vi "Color Wheel Controller.vi"(8 "error in":errorcluster) -> ()   [LabVIEW 2019]
doc: "This VI executes continuously carrying out the current operation and responding to updates or new operations. It will often contain the timing or control code that is difficult to place directly in TeleOp. This VI generally opens all sensors and motors and isolates the rest of the robot code from knowing how the operations are carried out."
uses:
  <vilib>/Rock Robotics/WPI/Framework/Completion Status.ctl
  Color Wheel Setpoints.ctl
  Color Wheel Operations.ctl
  <vilib>/Rock Robotics/WPI/ThirdParty/Phoenix-LabVIEW/Motor Controller/Controls/CTRE_Phoenix_MotorControl_ControlMode.ctl
  <vilib>/Rock Robotics/WPI/ThirdParty/Phoenix-LabVIEW/Motor Controller/Get/CTRE_Phoenix_MotorController_GetSelectedSensorData.vi
  <vilib>/Rock Robotics/Network Tables/NT Read Number.vi
  <vilib>/Rock Robotics/Network Tables/NT Write Boolean.vi
panel:
  in  "slotIdx":i32
  in  "Tx Red":dbl
  in  "Tx Blue":dbl
  in  "Tx Green":dbl
  in  "Tx Yellow":dbl
  in  "Ticks per full rotation":dbl
  out "Position (Raw Sensor Units)":i32
  in  "PIDF Constants":cluster{"P":dbl, "I":dbl, "D":dbl, "F":dbl}
  in  "Interactive Values":T1
  out "Current\nCmd":string
  in  "Buttons":cluster{"Execute Cmd":bool, "Abort Cmd":bool}
  out "Command Timing":cluster{"Start Time (ms)":u32, "Iterations":i32}
  out "Status":T3
  # "Tip: It may be helpful to observe inputs and sensor values.\nYou may also want to display tuning or debugging controls."
  # "Interactive Command: You may fill in the settings for a command\nand schedule it with the Execute button. You can observe and abort\nany command while fine tuning the code for the controller."
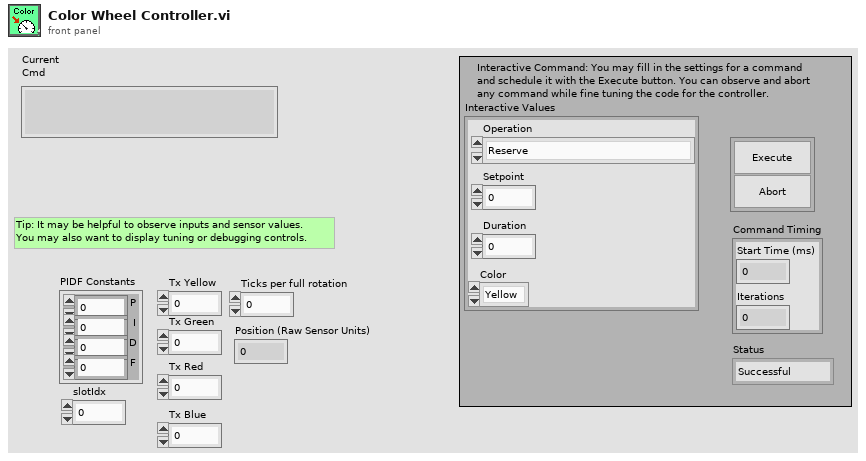
[diagram p1: front panel]
types:
  T1 = typedef "Color Wheel Setpoints.ctl" = cluster{"Operation":T2, "Setpoint":dbl, "Duration":dbl, "Color":enum16{"Yellow", "Green", "Blue", "Red"}}
  T2 = typedef "Color Wheel Operations.ctl" = enum16{"Reserve", "Read Current", "Immediate", "Rotation Control", "Position Control"}
  T3 = typedef "Completion Status.ctl" = enum16{"Successful", "Aborted", "Incomplete"}
  T4 = typedef "WPI_MotorControlDeviceRef.ctl" = cluster{"DeviceStatus":errorcluster, "Type":T5, "PWM":cluster{"PWM Channel":T6, "DeadBand":T7}, "CAN":cluster{"Device Number":u8, "SetOutput VI Ref":variant, "GetOutput VI Ref":variant, "Enable VI Ref":variant, "Disable VI Ref":variant, "Data":variant}, "Invert":bool, "DIO PWM":cluster{"PWM \"Enable\" Channel":T6, "DIOChannel":T8, "PWM Rate":dbl}}
  T5 = typedef "WPI_MotorControlType.ctl" = enum16{"PWM", "CAN", "DIO PWM"}
  T6 = typedef "FPGA_DIOPWMChannel.ctl" = enum8{"PWM 0", "PWM 1", "PWM 2", "PWM 3", "PWM 4", "PWM 5", "PWM 6", "PWM 7", "PWM 8", "PWM 9", "PWM MXP 0", "PWM MXP 1", "PWM MXP 2", "PWM MXP 3", "PWM MXP 4", "PWM MXP 5", "PWM MXP 6", "PWM MXP 7", "PWM MXP 8", "PWM MXP 9", "Invalid"}
  T7 = typedef "WPI_PWMDeadband.ctl" = cluster{"Name":string, "maxPositivePwm":i32, "minPositivePwm":i32, "centerPwm":i32, "maxNegativePwm":i32, "minNegativePwm":i32, "angularRange":u16}
  T8 = typedef "FPGA_DIOChannel.ctl" = enum8{"DIO 0", "DIO 1", "DIO 2", "DIO 3", "DIO 4", "DIO 5", "DIO 6", "DIO 7", "DIO 8", "DIO 9", "DIO MXP 0", "DIO MXP 1", "DIO MXP 2", "DIO MXP 3", "DIO MXP 4", "DIO MXP 5", "DIO MXP 6", "DIO MXP 7", "DIO MXP 8", "DIO MXP 9", "DIO MXP 10", "DIO MXP 11", "DIO MXP 12", "DIO MXP 13", "DIO MXP 14", "DIO MXP 15", "SPI Port CS1", "SPI Port CS2", "SPI Port CS3", "SPI Port MISO", "SPI Port MOSI", "Invalid"}
  T9 = typedef "Command Status Info.ctl" = cluster{"Name":string, "Status":T3, "notifier out":T10}
  T10 = typedef "Completion Notifier.ctl" = refnum<notifier>
  T11 = cluster{"Current Command":T1, "Command Timing":cluster{"Start Time (ms)":u32, "Iterations":i32}, "Command Arguments":cluster{"Command Info":T9, "Description":string, "Default Command":T1, "queue out":refnum<queue>, "Subsystem Name":string}}
  T12 = typedef "CTRE_Phoenix_MotorControl_ControlMode.ctl" = u16
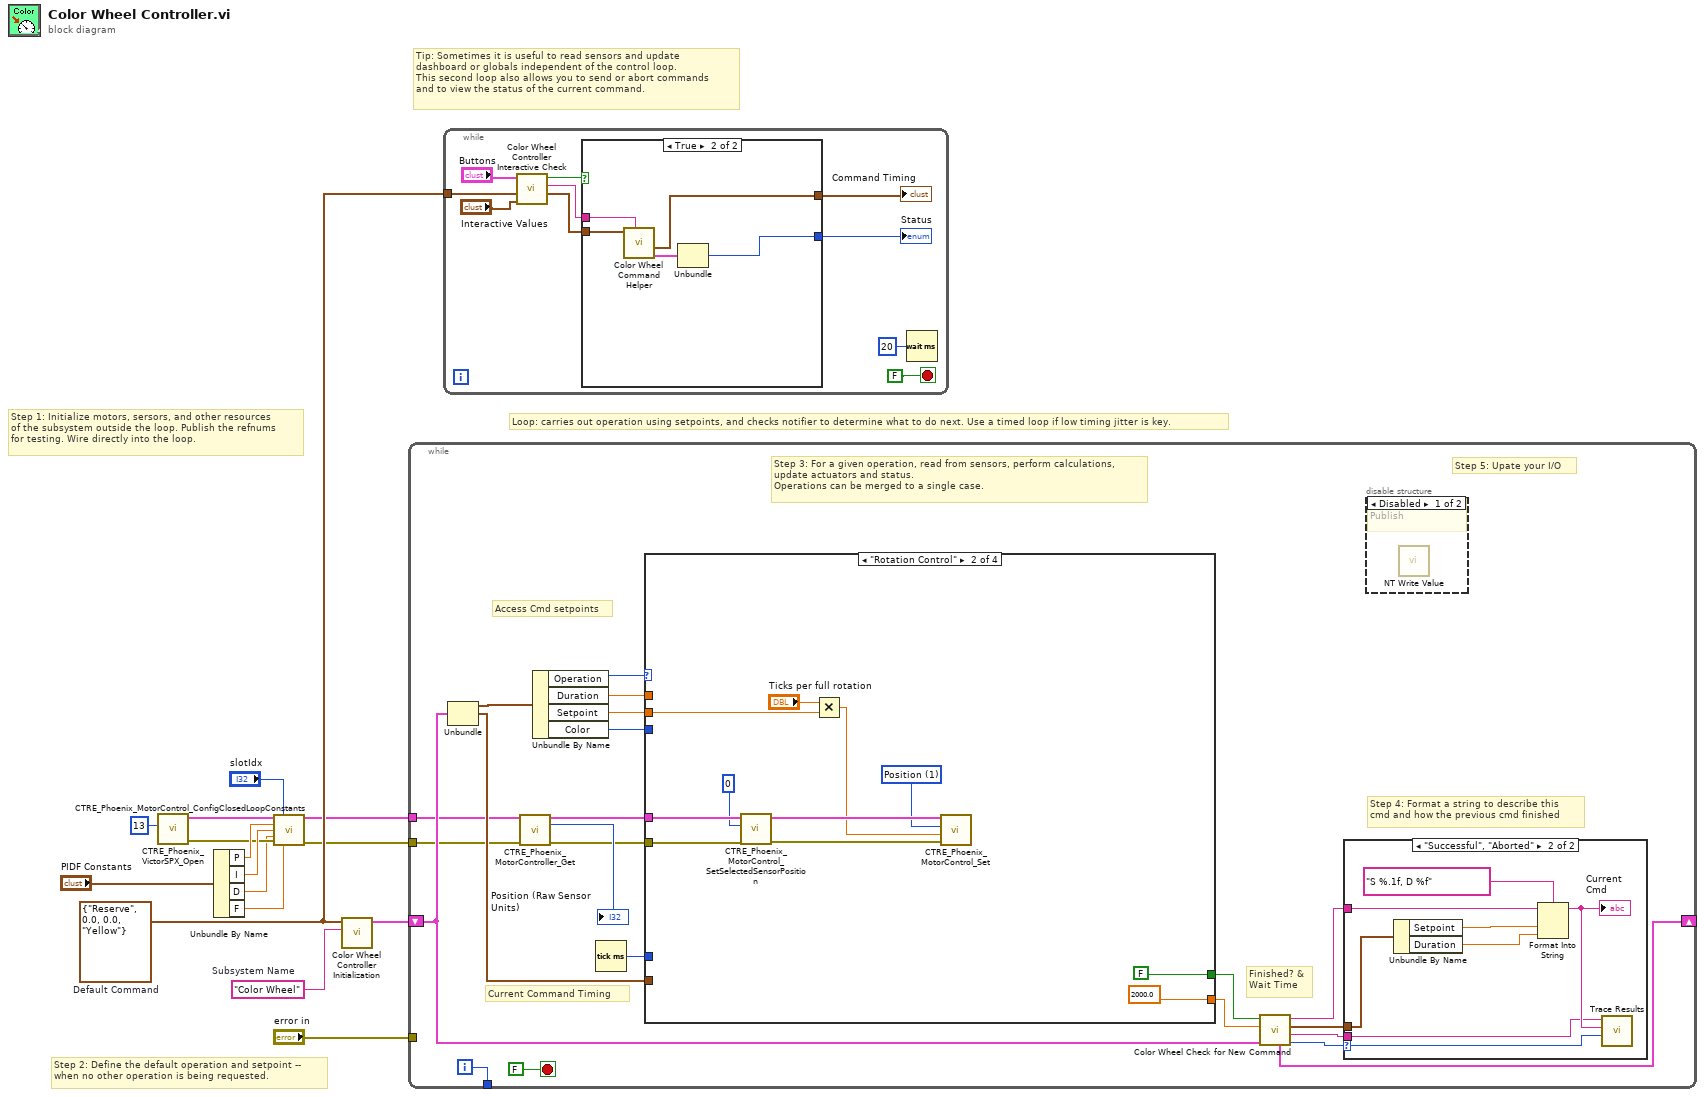
[diagram p0: block diagram]
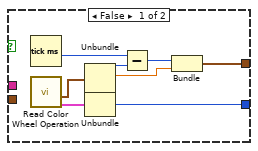
[diagram p2: hidden frame]
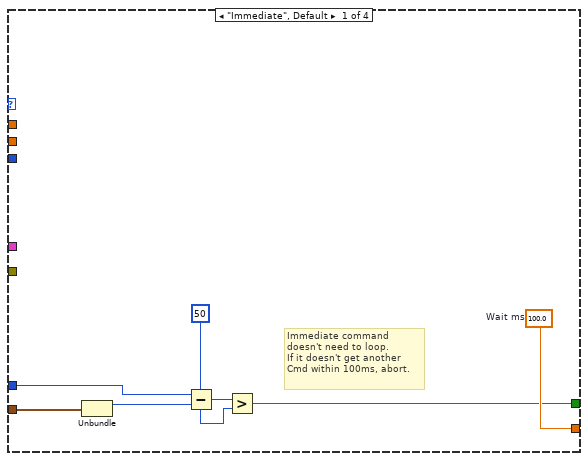
[diagram p5: hidden frame]
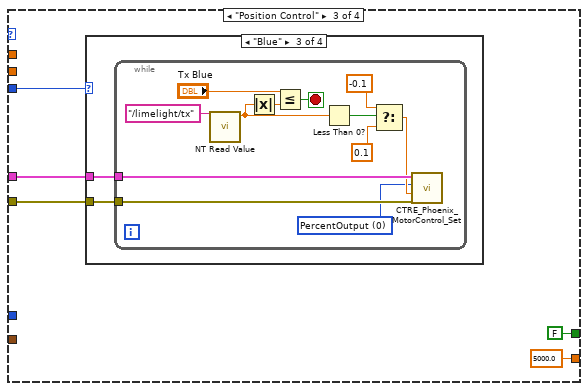
[diagram p6: hidden frame]
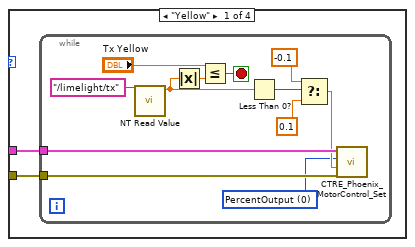
[diagram p7: hidden frame]
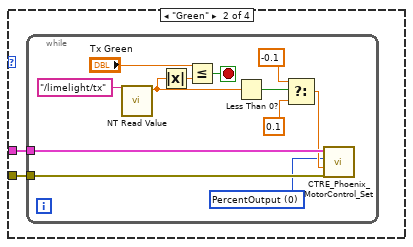
[diagram p8: hidden frame]
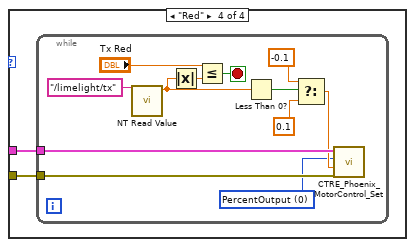
[diagram p9: hidden frame]
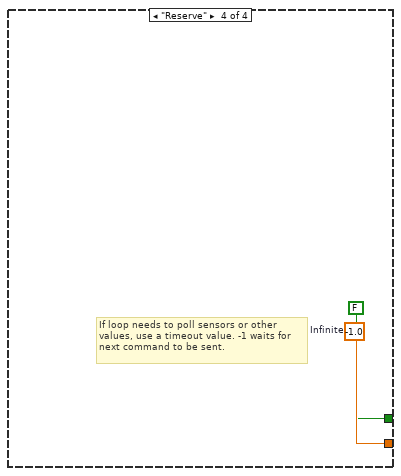
[diagram p10: hidden frame]
diagram:
  w9 = T1 {"Operation"=enum."Reserve", "Setpoint"=0.0, "Duration"=0.0, "Color"=enum."Yellow"}  # Default Command
  w13 = "Color Wheel"  # Subsystem Name
  # "Tip: Sometimes it is useful to read sensors and update\ndashboard or globals independent of the control loop.\nThis second loop also allows you to send or abort commands\nand to view the status of the current command."
  # "Step 2: Define the default operation and setpoint --\nwhen no other operation is being requested."
  # "Step 1: Initialize motors, sersors, and other resources\nof the subsystem outside the loop. Publish the refnums\nfor testing. Wire directly into the loop."
  # "Loop: carries out operation using setpoints, and checks notifier to determine what to do next. Use a timed loop if low timing jitter is key."
  n1 = call <vilib>:"CTRE_Phoenix_VictorSPX_Open.vi"("Device Number"=u8 13) -> ("error out"=w5:errorcluster, "CAN Talon SRX Ref"=w11:T4)  [unwired: 9 in]
  n2 = Unbundle By Name("PIDF Constants") -> ("P"=w8:dbl, "I"=w7:dbl, "D"=w2:dbl, "F"=w6:dbl)
  n3 = call <vilib>:"CTRE_Phoenix_MotorControl_ConfigClosedLoopConstants.vi"("PhoenixMotorControlDevRef"=w11, "slotIdx"="slotIdx", "P"=w8, "I"=w7, "D"=w2, "error in (no error)"=w5, "F"=w6) -> ("PhoenixMotorControlDevRef"=w4:T4, "error out"=w3:errorcluster)  [unwired: 7 in]
  n4 = call "Color Wheel Controller Initialization.vi"("Subsystem Name"=w13, "Default Command"=w9) -> ("Current Command"=w14:T11)  [unwired: 9 in]
  n5 = while {
    shift-right: [w29] -> _
    shift-left: w14 -> [w22]
    tunnel: [w36] -> _
    tunnel: "error in" -> [_]
    tunnel: w4 -> [w21]
    tunnel: w3 -> [w20]
    i -> [w36]
    stop <- FALSE stop-if-true
    # "Step 5: Upate your I/O"
    # "Step 4: Format a string to describe this\ncmd and how the previous cmd finished"
    # "Current Command Timing"
    # "Access Cmd setpoints"
    # "Finished? &\nWait Time"
    # "Step 3: For a given operation, read from sensors, perform calculations,\nupdate actuators and status.\nOperations can be merged to a single case."
    n6 = Unbundle(w22) -> ("Current Command"=w35:T1, "Command Timing"=w31:cluster{"Start Time (ms)":u32, "Iterations":i32})  [unwired: 1 out]
    n7 = call-poly <vilib>:"CTRE_Phoenix_MotorController_Get.vi"("PhoenixMotorControlDevRef"=w21, "error in"=w20) -> ("PhoenixMotorControlDevRef"=w17:T4, "Position (Raw Sensor Units)"=→"Position (Raw Sensor Units)":i32, "error out"=w18:errorcluster)  [unwired: 10 in, 1 out]
    n8 = Unbundle By Name(w35) -> ("Operation"=w34:T2, "Duration"=w33:dbl, "Setpoint"=w30:dbl, "Color"=w16:enum16{"Yellow", "Green", "Blue", "Red"})
    n9 = Tick Count (ms)() -> (millisecond timer value=w32:u32)
    n10 = case shown="\"Rotation Control\"" w34 {
      tunnel: [w52 2000.0 ("Infinite") 5000.0 ("Infinite") w126] -> w27
      tunnel: [w46 FALSE ("ignore previous (F)") FALSE ("ignore previous (F)") FALSE ("ignore previous (F)")] -> w28
      tunnel: w31 -> [w48 _ _ _]
      tunnel: w33 -> [_ _ _ _]
      tunnel: w32 -> [w47 _ _ _]
      tunnel: w30 -> [_ w54 _ _]
      tunnel: w17 -> [_ w63 w67 _]
      tunnel: w18 -> [_ w61 w66 _]
      tunnel: w16 -> [_ _ w68 _]
      frame "Immediate", Default {
        w52 = 100.0  # Wait ms
        # "Immediate command\ndoesn't need to loop.\nIf it doesn't get another\nCmd within 100ms, abort."
        n11 = Unbundle(w48) -> ("Start Time (ms)"=w51:u32)  [unwired: 1 out]
        n12 = Subtract(x=w47, y=w51) -> (x-y=w50:u32)
        n13 = Greater?(x=w50, y=u8 50 ("Left Motor")) -> (0:w46:bool)
      }
      frame "Rotation Control" {
        w55 = T12 1 items=["PercentOutput"=0, "Position"=1, "Velocity"=2, "Current"=3, "Follower"=5, "MotionProfile"=6, "MotionMagic"=7, "MotionProfileArc"=10, "Disabled"=15] ("Control Mode")
        n14 = call <vilib>:"CTRE_Phoenix_MotorControl_SetSelectedSensorPosition.vi"("error in (no error)"=w61, "New Sensor Position"=0, "PhoenixMotorControlDevRef"=w63) -> ("error out"=w57:errorcluster, "PhoenixMotorControlDevRef"=w58:T4)  [unwired: 7 in]
        n15 = Multiply(x="Ticks per full rotation", y=w54) -> (x*y=w56:dbl)
        n16 = call <vilib>:"CTRE_Phoenix_MotorControl_Set.vi"("error in (no error)"=w57, "Output"=w56, "Control Mode"=w55, "PhoenixMotorControlDevRef"=w58) -> ()  [unwired: 6 in, 2 out]
      }
      frame "Position Control" {
        n17 = case shown="\"Blue\"" w68 {
          tunnel: w67 -> [w70 w84 w98 w112]
          tunnel: w66 -> [w69 w83 w97 w111]
          frame "Yellow" {
            n18 = while {
              tunnel: w70 -> [w78]
              tunnel: w69 -> [w77]
              stop <- w72 stop-if-true
              w75 = T12 0 items=["PercentOutput"=0, "Position"=1, "Velocity"=2, "Current"=3, "Follower"=5, "MotionProfile"=6, "MotionMagic"=7, "MotionProfileArc"=10, "Disabled"=15] ("Control Mode")
              n19 = call-poly <vilib>:"NT Read Value.vi"("Name"="/limelight/tx") -> ("Numeric"=w73:dbl)  [unwired: 9 in, 1 out]
              n20 = Absolute Value(x=w73) -> (abs(x)=w74:dbl)
              n21 = Less Or Equal?(x="Tx Yellow", y=w74) -> (x <= y?=w72:bool)
              n22 = Less Than 0?(x=w73) -> (x < 0?=w81:bool)
              n23 = Select(t=-0.1, s=w81, f=0.1) -> (s? t:f=w76:dbl)
              n24 = call <vilib>:"CTRE_Phoenix_MotorControl_Set.vi"("error in (no error)"=w77, "Output"=w76, "Control Mode"=w75, "PhoenixMotorControlDevRef"=w78) -> ()  [unwired: 6 in, 2 out]
            }
          }
          frame "Green" {
            n25 = while {
              tunnel: w84 -> [w92]
              tunnel: w83 -> [w91]
              stop <- w86 stop-if-true
              w89 = T12 0 items=["PercentOutput"=0, "Position"=1, "Velocity"=2, "Current"=3, "Follower"=5, "MotionProfile"=6, "MotionMagic"=7, "MotionProfileArc"=10, "Disabled"=15] ("Control Mode")
              n26 = call-poly <vilib>:"NT Read Value.vi"("Name"="/limelight/tx") -> ("Numeric"=w87:dbl)  [unwired: 9 in, 1 out]
              n27 = Absolute Value(x=w87) -> (abs(x)=w88:dbl)
              n28 = Less Or Equal?(x="Tx Green", y=w88) -> (x <= y?=w86:bool)
              n29 = Less Than 0?(x=w87) -> (x < 0?=w95:bool)
              n30 = Select(t=-0.1, s=w95, f=0.1) -> (s? t:f=w90:dbl)
              n31 = call <vilib>:"CTRE_Phoenix_MotorControl_Set.vi"("error in (no error)"=w91, "Output"=w90, "Control Mode"=w89, "PhoenixMotorControlDevRef"=w92) -> ()  [unwired: 6 in, 2 out]
            }
          }
          frame "Blue" {
            n32 = while {
              tunnel: w98 -> [w106]
              tunnel: w97 -> [w105]
              stop <- w100 stop-if-true
              w103 = T12 0 items=["PercentOutput"=0, "Position"=1, "Velocity"=2, "Current"=3, "Follower"=5, "MotionProfile"=6, "MotionMagic"=7, "MotionProfileArc"=10, "Disabled"=15] ("Control Mode")
              n33 = call-poly <vilib>:"NT Read Value.vi"("Name"="/limelight/tx") -> ("Numeric"=w101:dbl)  [unwired: 9 in, 1 out]
              n34 = Absolute Value(x=w101) -> (abs(x)=w102:dbl)
              n35 = Less Or Equal?(x="Tx Blue", y=w102) -> (x <= y?=w100:bool)
              n36 = Less Than 0?(x=w101) -> (x < 0?=w109:bool)
              n37 = Select(t=-0.1, s=w109, f=0.1) -> (s? t:f=w104:dbl)
              n38 = call <vilib>:"CTRE_Phoenix_MotorControl_Set.vi"("error in (no error)"=w105, "Output"=w104, "Control Mode"=w103, "PhoenixMotorControlDevRef"=w106) -> ()  [unwired: 6 in, 2 out]
            }
          }
          frame "Red" {
            n39 = while {
              tunnel: w112 -> [w120]
              tunnel: w111 -> [w119]
              stop <- w114 stop-if-true
              w117 = T12 0 items=["PercentOutput"=0, "Position"=1, "Velocity"=2, "Current"=3, "Follower"=5, "MotionProfile"=6, "MotionMagic"=7, "MotionProfileArc"=10, "Disabled"=15] ("Control Mode")
              n40 = call-poly <vilib>:"NT Read Value.vi"("Name"="/limelight/tx") -> ("Numeric"=w115:dbl)  [unwired: 9 in, 1 out]
              n41 = Absolute Value(x=w115) -> (abs(x)=w116:dbl)
              n42 = Less Or Equal?(x="Tx Red", y=w116) -> (x <= y?=w114:bool)
              n43 = Less Than 0?(x=w115) -> (x < 0?=w123:bool)
              n44 = Select(t=-0.1, s=w123, f=0.1) -> (s? t:f=w118:dbl)
              n45 = call <vilib>:"CTRE_Phoenix_MotorControl_Set.vi"("error in (no error)"=w119, "Output"=w118, "Control Mode"=w117, "PhoenixMotorControlDevRef"=w120) -> ()  [unwired: 6 in, 2 out]
            }
          }
        }
      }
      frame "Reserve" {
        w126 = -1.0  # Infinite
        # "If loop needs to poll sensors or other\nvalues, use a timeout value. -1 waits for\nnext command to be sent."
      }
    }
    n46 = call "Color Wheel Check for New Command.vi"("Current Command"=w22, "Wait time (ms)"=w27, "Finished?"=w28) -> ("Completion"=w23:T3, "Subsystem Name"=w24:string, "Current Command"=w25:T1, "Initial Trace String"=w26:string, "NextCommand"=w29:T11)  [unwired: 4 in]
    n47 = case shown="\"Successful\", \"Aborted\"" w23 {
      selector: w23 -> [_ w45]
      tunnel: w26 -> [_ w41]
      tunnel: w25 -> [_ w42]
      tunnel: w24 -> [_ w38]
      frame "Incomplete", Default {
        # "Continuing current command"
      }
      frame "Successful", "Aborted" {
        # "Report and setup for next command"
        n48 = Unbundle By Name(w42) -> ("Setpoint"=w44:dbl, "Duration"=w39:dbl)
        n49 = Format Into String(format string="S %.1f, D %f", initial string=w41, w44, w39) -> (resulting string=w40:string)  [unwired: 1 in, 1 out]
        "Current\nCmd" <- w40
        n50 = call <vilib>:"Trace Results.vi"("Status of previous command"=w45, "Description"=w40, "Subsystem"=w38) -> ()  [unwired: 9 in]
      }
    }
    n51 = disable-structure shown="Disabled" {
      frame Disabled {
        # "Publish"
        n52 = call-poly <vilib>:"NT Write Value.vi"() -> ()  [unwired: 11 in, 1 out]
      }
      frame Enabled {
      }
    }
  }
  n53 = while {
    tunnel: w9 -> [w133]
    stop <- FALSE stop-if-true
    n54 = call "Color Wheel Controller Interactive Check.vi"("Interactive Command in"="Interactive Values", "Default Command"=w133, "Buttons"="Buttons") -> ("Interactive Command out"=w130:T1, "Trace String"=w131:string, "Schedule"=w132:bool)  [unwired: 6 in]
    n55 = case shown="True" w132 {
      tunnel: [w144 w149] -> w129
      tunnel: w130 -> [_ w147]
      tunnel: [w140 w145] -> w128
      tunnel: w131 -> [_ w148]
      frame False {
        n56 = Tick Count (ms)() -> (millisecond timer value=w139:u32)
        n57 = call "Read Color Wheel Operation.vi"() -> ("Command Info"=w137:T9, "SubSystem Data"=w138:T1)  [unwired: 9 in, 1 out]
        n58 = Unbundle(w138) -> ("Operation"=w143:T2, "Setpoint"=w141:dbl)  [unwired: 2 out]
        n59 = Unbundle(w137) -> ("Status"=w144:T3)  [unwired: 2 out]
        n60 = Subtract(x=w139, y=w143) -> (x-y=w142:u32)
        n61 = Bundle(w142, "Setpoint"=w141) -> (w140:cluster{u32, "Setpoint":dbl})  [unwired: 1 in]
      }
      frame True {
        n62 = call "Color Wheel Command Helper.vi"("Description"=w148, "SubSystem Data"=w147) -> ("Command Info Out"=w146:T9, "Command Timing"=w145:cluster{"Start Time (ms)":u32, "Iterations":i32})  [unwired: 7 in, 1 out]
        n63 = Unbundle(w146) -> ("Status"=w149:T3)  [unwired: 2 out]
      }
    }
    "Status" <- w129
    "Command Timing" <- w128
    n64 = Wait (ms)(milliseconds to wait=u32 20) -> ()  [unwired: 1 out]
  }
